vi "RTS Calculate Chamber CoolDehum Temps.vi"(8 "Error In":errorcluster, 11 "Room Setpoints":T1={"Room Setpoint Temperature (*RM Dry Set P1)"=90.0, "Room Setpoint Humidity (*RM Hum Set P1)"=20.0, "Room Cool Temperature (*RM Cool Setp 1)"=65.0, "Room Dehum Temperature (*RM De Hum Set P1)"=60.0} {"Room Dehum Temperature (*RM De Hum Set P1)" min=30.0 max=120.0; "Room Cool Temperature (*RM Cool Setp 1)" min=30.0 max=120.0; "Room Setpoint Humidity (*RM Hum Set P1)" min=5.0 max=98.0; "Room Setpoint Temperature (*RM Dry Set P1)" min=40.0 max=120.0}) -> (0 "Error Out":errorcluster, 3 "Room Setpoint Output":T1={"Room Setpoint Temperature (*RM Dry Set P1)"=90.0, "Room Setpoint Humidity (*RM Hum Set P1)"=20.0, "Room Cool Temperature (*RM Cool Setp 1)"=65.0, "Room Dehum Temperature (*RM De Hum Set P1)"=60.0} {"Room Dehum Temperature (*RM De Hum Set P1)" min=30.0 max=120.0; "Room Cool Temperature (*RM Cool Setp 1)" min=30.0 max=120.0; "Room Setpoint Humidity (*RM Hum Set P1)" min=5.0 max=98.0; "Room Setpoint Temperature (*RM Dry Set P1)" min=40.0 max=120.0})   [LabVIEW 2016]
uses:
  Type Definitions/RTS Chamber Temperature Humidity Control.ctl
  <vilib>/Analysis/NI_AALPro.lvlib
panel:
  out "Cool Temp":dbl[](array[numeric])
  out "x/y":dbl[](array[numeric])
  out "Polynomial Coefficients":dbl[](array[numeric])
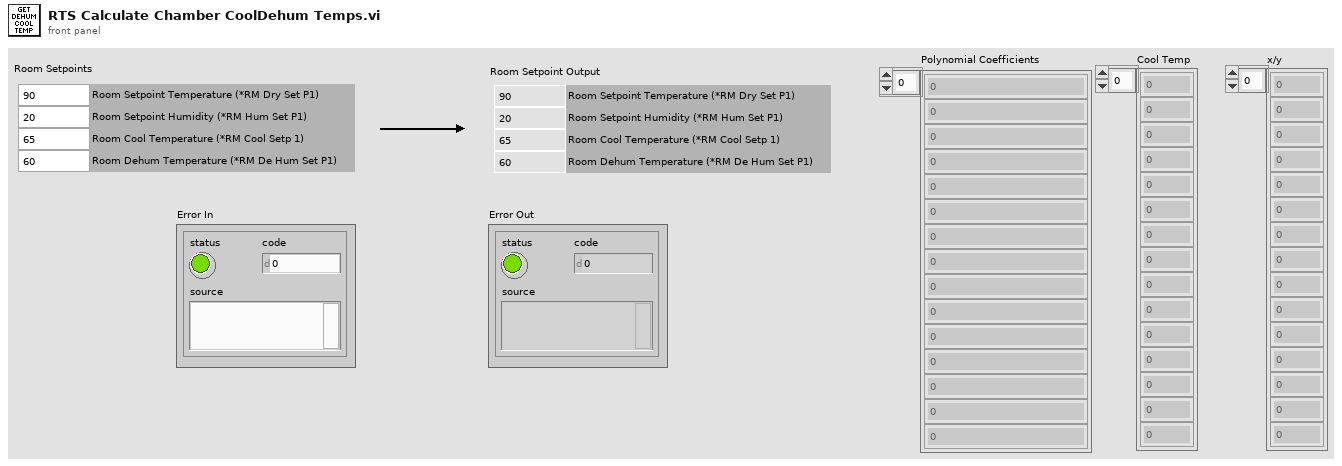
[diagram p1: front panel]
types:
  T1 = typedef "RTS Chamber Temperature Humidity Control.ctl" = cluster{"Room Setpoint Temperature (*RM Dry Set P1)":dbl, "Room Setpoint Humidity (*RM Hum Set P1)":dbl, "Room Cool Temperature (*RM Cool Setp 1)":dbl, "Room Dehum Temperature (*RM De Hum Set P1)":dbl}
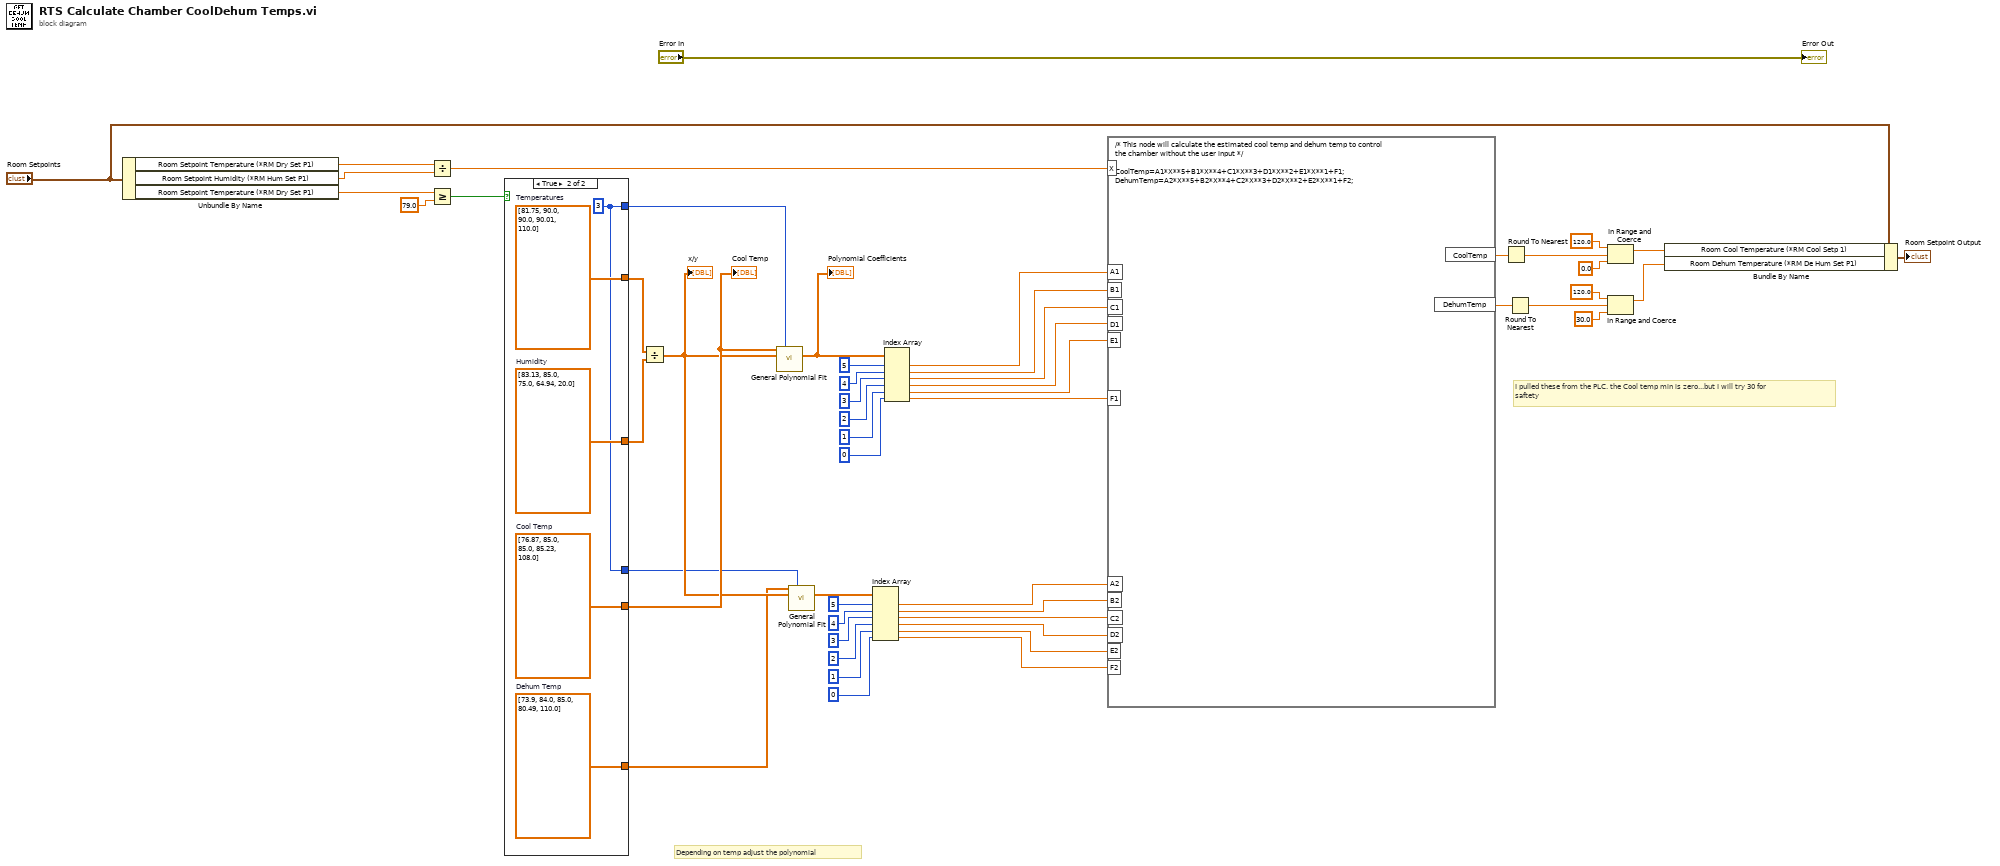
[diagram p0: block diagram]
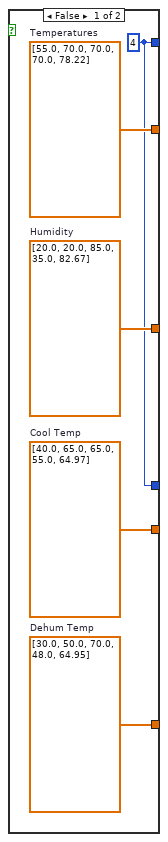
[diagram p2: hidden frame]
diagram:
  # "Depending on temp adjust the polynomial"
  # "I pulled these from the PLC. the Cool temp min is zero...but I will try 30 for\nsaftety"
  n1 = Unbundle By Name("Room Setpoints") -> ("Room Setpoint Temperature (*RM Dry Set P1)"=w52:dbl, "Room Setpoint Humidity (*RM Hum Set P1)"=w51:dbl, "Room Setpoint Temperature (*RM Dry Set P1)"=w32:dbl)
  n2 = Divide(x=w52, y=w51) -> (x/y=w50:dbl)
  n3 = Greater Or Equal?(x=w32, y=79.0) -> (x >= y?=w11:bool)
  n4 = case shown="True" w11 {
    tunnel: [w57 w62] -> w30
    tunnel: [w56 w61] -> w29
    tunnel: [w55 w60] -> w28
    tunnel: [w54 w59] -> w26
    tunnel: [w53 w58] -> w10
    tunnel: [w53 w58] -> w9
    frame False {
      w53 = 4 ("polynomial order")
      w54 = dbl[] [30.0, 50.0, 70.0, 48.0, 64.95]  # Dehum Temp
      w55 = dbl[] [40.0, 65.0, 65.0, 55.0, 64.97]  # Cool Temp
      w56 = dbl[] [20.0, 20.0, 85.0, 35.0, 82.67]  # Humidity
      w57 = dbl[] [55.0, 70.0, 70.0, 70.0, 78.22]  # Temperatures
    }
    frame True {
      w58 = 3 ("polynomial order")
      w59 = dbl[] [73.9, 84.0, 85.0, 80.49, 110.0]  # Dehum Temp
      w60 = dbl[] [76.87, 85.0, 85.0, 85.23, 108.0]  # Cool Temp
      w61 = dbl[] [83.13, 85.0, 75.0, 64.94, 20.0]  # Humidity
      w62 = dbl[] [81.75, 90.0, 90.0, 90.01, 110.0]  # Temperatures
    }
  }
  "Cool Temp" <- w28
  n5 = Divide(x=w30, y=w29) -> (x/y=w27:dbl[])
  "x/y" <- w27
  n6 = call <vilib>:"General Polynomial Fit.vi"("Y"=w28, "polynomial order"=w10, "X"=w27) -> ("Polynomial Coefficients"=w25:dbl[])  [unwired: 9 in, 3 out]
  "Polynomial Coefficients" <- w25
  n7 = call <vilib>:"General Polynomial Fit.vi"("Y"=w26, "polynomial order"=w9, "X"=w27) -> ("Polynomial Coefficients"=w12:dbl[])  [unwired: 9 in, 3 out]
  n8 = Index Array(array=w12, index #1=5 ("index"), index #2=4 ("index"), index #3=3 ("index"), index #4=2 ("index"), index #5=1 ("index"), index #6=0 ("index")) -> (element #1=w43:dbl, element #2=w42:dbl, element #3=w41:dbl, element #4=w40:dbl, element #5=w39:dbl, element #6=w38:dbl)
  n9 = Index Array(array=w25, index #1=5 ("index"), index #2=4 ("index"), index #3=3 ("index"), index #4=2 ("index"), index #5=1 ("index"), index #6=0 ("index")) -> (element #1=w49:dbl, element #2=w48:dbl, element #3=w47:dbl, element #4=w46:dbl, element #5=w45:dbl, element #6=w44:dbl)
  n10 = formula code="/* This node will calculate the estimated cool temp and dehum temp to control\nthe chamber without the user input */\n\nCoolTemp=A1*X**5+B1*X**4+C1*X**3+D1*X**2+E1*X**1+F1;\nDehumTemp=A2*X**5+B2*X**4+C2*X**3+D2*X**2+E2*X**1+F2;"("X"=w50, "A1"=w49, "B1"=w48, "C1"=w47, "D1"=w46, "E1"=w45, "F1"=w44, "A2"=w43, "B2"=w42, "C2"=w41, "D2"=w40, "E2"=w39, "F2"=w38) -> ("CoolTemp"=w36:dbl, "DehumTemp"=w37:dbl)
  n11 = Round To Nearest(number=w36) -> (nearest integer value=w8:dbl)
  n12 = Round To Nearest(number=w37) -> (nearest integer value=w2:dbl)
  n13 = In Range and Coerce(upper limit=120.0, x=w8, lower limit=0.0) -> (coerced(x)=w5:dbl)  [unwired: 1 out]
  n14 = In Range and Coerce(upper limit=120.0, x=w2, lower limit=30.0) -> (coerced(x)=w1:dbl)  [unwired: 1 out]
  n15 = Bundle By Name(cluster="Room Setpoints", "Room Cool Temperature (*RM Cool Setp 1)"=w5, "Room Dehum Temperature (*RM De Hum Set P1)"=w1) -> (→"Room Setpoint Output":T1)
  "Error Out" <- "Error In"
